vi "Set Image.vi"(0 "image in":refnum<class "MSC Image.lvclass">, 1 "Image":T1 {"Image Type" items=["Grayscale U8"=0, "Grayscale U16"=2, "Grayscale Single"=5, "Grayscale Double"=6, "RGB U8"=16]}, 5 "error in (no error)":errorcluster) -> (14 "image out":refnum<class "MSC Image.lvclass">, 19 "error out":errorcluster)   [LabVIEW 2014, in "MSC Image.lvclass"]
doc: "Interface to any other software."
uses:
  MSC Image.lvclass
  controls/Image.ctl
  controls/Size.ctl
  controls/Image Type.ctl
  MSC Image.lvclass/MSC Image.ctl
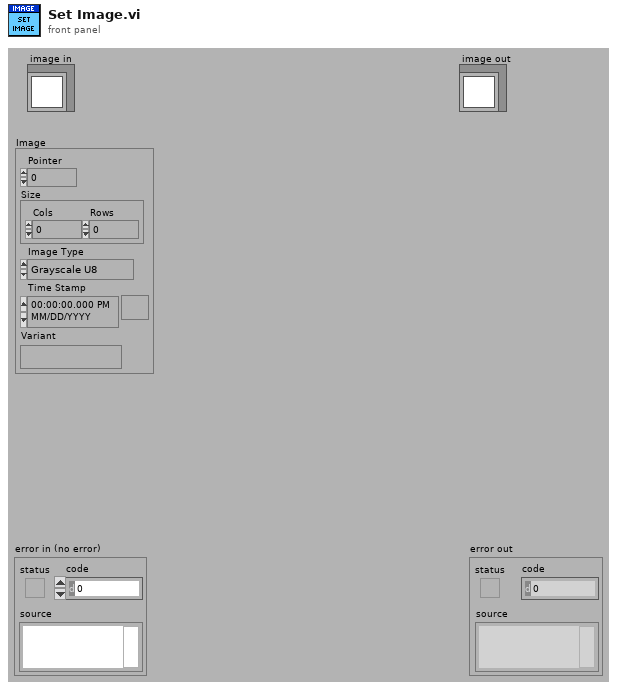
[diagram p1: front panel]
types:
  T1 = typedef "MSC Image.lvclass/Image.ctl" = cluster{"Pointer":u64, "Size":T2, "Image Type":T3, "Time Stamp":timestamp, "Variant":variant}
  T2 = typedef "MSC Image.lvclass/Size.ctl" = cluster{"Cols":i32, "Rows":i32}
  T3 = typedef "MSC Image.lvclass/Image Type.ctl" = i32
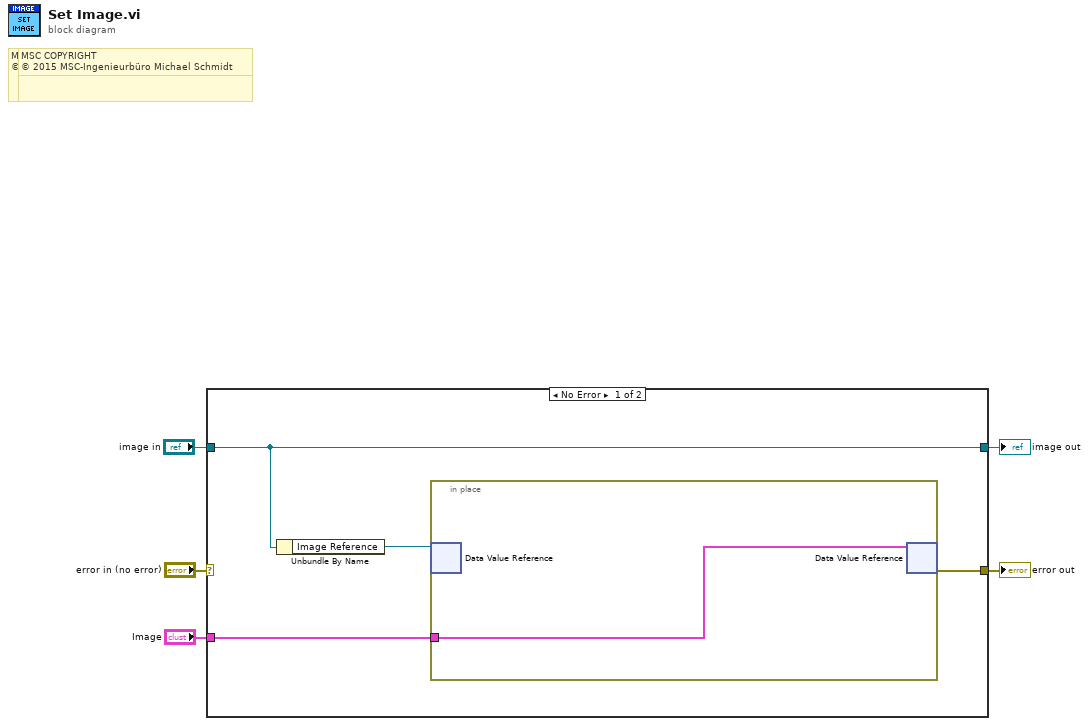
[diagram p0: block diagram]
diagram:
  # "MSC COPYRIGHT\n© 2016 MSC-Ingenieurbüro Michael Schmidt"
  # "MSC COPYRIGHT\n© 2016 MSC-Ingenieurbüro Michael Schmidt"
  # "MSC COPYRIGHT\n© 2015 MSC-Ingenieurbüro Michael Schmidt"
  # "MSC COPYRIGHT\n© 2015 MSC-Ingenieurbüro Michael Schmidt"
  n1 = case shown="No Error" "error in (no error)" {
    selector: "error in (no error)" -> [_ w12]
    tunnel: [w6 w12] -> w4
    tunnel: [w8 w11] -> w2
    tunnel: "image in" -> [w8 w11]
    tunnel: "Image" -> [w7 _]
    frame No Error {
      n2 = Unbundle By Name(w8) -> ("Image Reference"=w9:refnum<data-value>)
      n3 = in-place {
        in-place-border: w7 -> [w10]
        n4 = in-place-dvr #1(w9) -> ()  [unwired: 2 out]
        n5 = in-place-dvr #1(w10) -> (w6:errorcluster)  [unwired: 1 out]
      }
    }
    frame Error {
    }
  }
  "error out" <- w4
  "image out" <- w2
